vi "find insert point.vi"(10 "string to insert":string, 11 "sorted strings":string[](array[string])) -> (3 "index":i32)   [LabVIEW 2013, in "tag bus.lvlib" / "binary search.lvlib"]
doc: "performs a binary search on the input array to find the location to insert an element. It <b>assumes</b> that the input list is sorted and the string to search for is not empty."
uses:
  binary search.lvlib
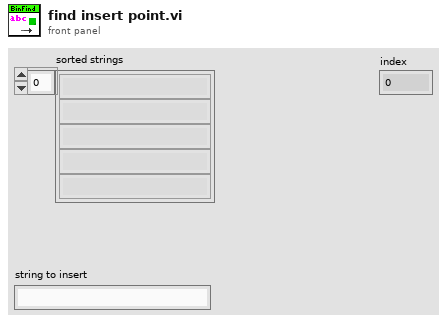
[diagram p1: front panel]
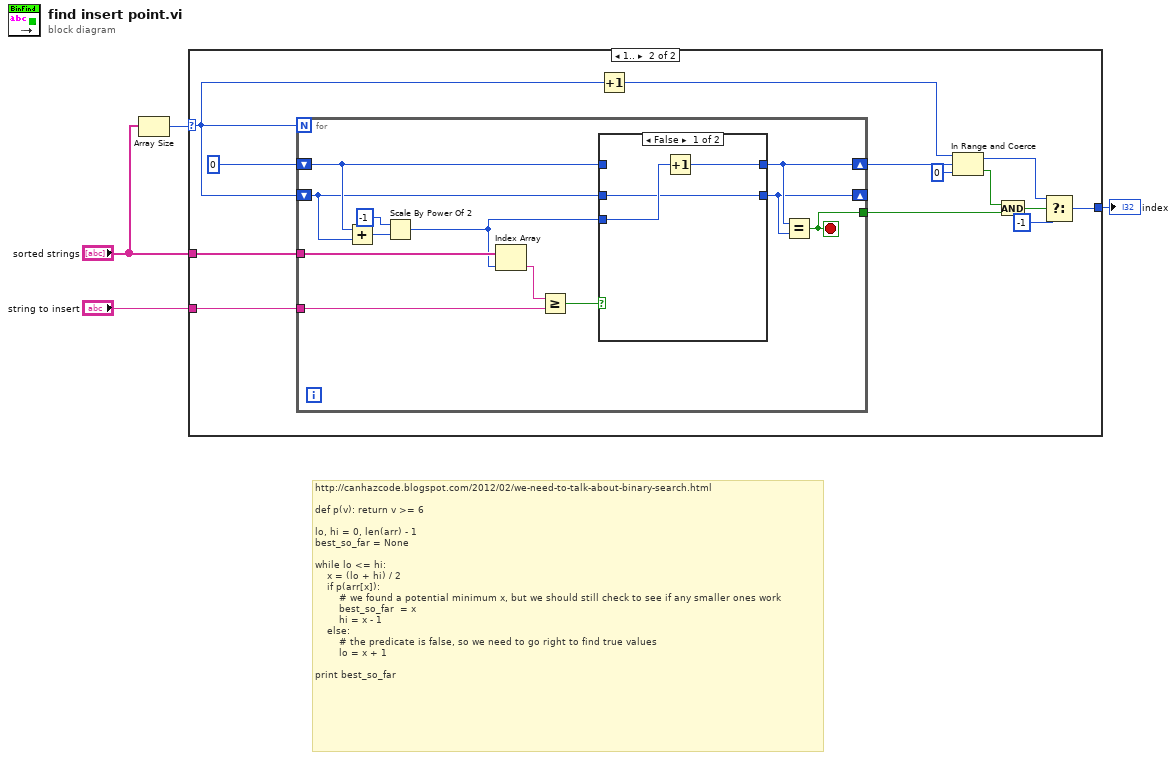
[diagram p0: block diagram]
diagram:
  # "http://canhazcode.blogspot.com/2012/02/we-need-to-talk-about-binary-search.html\n\ndef p(v): return v >= 6\n \nlo, hi = 0, len(arr) - 1\nbest_so_far = None\n \nwhile lo <= hi:\n    x = (lo + hi) / 2\n    if p(arr[x]):\n        # we found a potential minimum x, but we should still check to see if any smaller ones work\n        best_so_far  = x\n        hi = x - 1\n    else:\n        # the predicate is false, so we need to go right to find true values\n        lo = x + 1\n \nprint best_so_far"
  n1 = Array Size(array="sorted strings") -> (size(s)=w1:i32)
  n2 = case shown="1.." w1 {
    selector: w1 -> [w5 w6]
    tunnel: "sorted strings" -> [_ w17]
    tunnel: "string to insert" -> [_ w16]
    tunnel: [w5 w8] -> w2
    frame 0, Default {
    }
    frame 1.. {
      n3 = for {
        N: w6 -> [_]
        shift-right: [w20] -> _
        shift-left: w6 -> [w22]
        shift-right: [w21] -> w15
        shift-left: 0 -> [w23]
        tunnel: w17 -> [w28]
        tunnel: w16 -> [w26]
        tunnel: [w19] -> w13
        stop <- w19 stop-if-true
        n4 = Add(x=w23, y=w22) -> (x+y=w30:i32)
        n5 = Scale By Power Of 2(n=i16 -1, x=w30) -> (x*2^n=w24:i32)
        n6 = Index Array(array=w28, index=w24) -> (element=w25:string)
        n7 = Greater Or Equal?(x=w25, y=w26) -> (x >= y?=w27:bool)
        n8 = case shown="False" w27 {
          tunnel: w24 -> [w33 w35]
          tunnel: w23 -> [_ w34]
          tunnel: w22 -> [w31 _]
          tunnel: [w32 w34] -> w21
          tunnel: [w31 w35] -> w20
          frame False {
            n9 = Increment(x=w33) -> (x+1=w32:i32)
          }
          frame True {
          }
        }
        n10 = Equal?(x=w21, y=w20) -> (x = y?=w19:bool)
      }
      n11 = Increment(x=w6) -> (x+1=w7:i32)
      n12 = In Range and Coerce(upper limit=w7, x=w15, lower limit=0) -> (coerced(x)=w10:i32, In Range?=w12:bool)
      n13 = And(x=w12, y=w13) -> (x .and. y?=w11:bool)
      n14 = Select(t=w10, s=w11, f=-1) -> (s? t:f=w8:i32)
    }
  }
  "index" <- w2
